vi "Create.vi"(8 "error in (no error)":errorcluster, 11 "NotifierMessenger in":refnum<class "NotifierMessenger.lvclass">) -> (0 "error out":errorcluster, 3 "NotifierMessenger out":refnum<class "NotifierMessenger.lvclass">)   [LabVIEW 2011, in "Messenging.lvlib" / "NotifierMessenger.lvclass"]
uses:
  NotifierMessenger.lvclass
  TextVarientMessage/MSG.lvclass
  NotifierMessenger.lvclass/NotifierMessenger.ctl
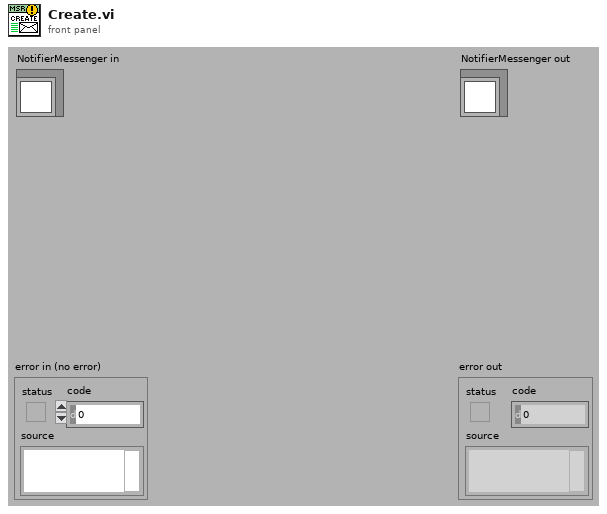
[diagram p1: front panel]
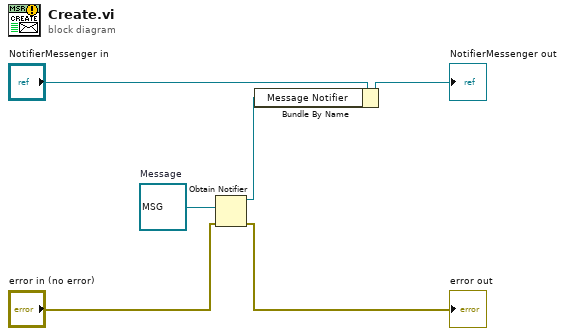
[diagram p0: block diagram]
diagram:
  w6 = refnum<class "MSG.lvclass"> refnum  # Message
  n1 = Obtain Notifier(notification data type=w6, error in (no error)="error in (no error)") -> (notifier out=w3:refnum<notifier>, error out=→"error out":errorcluster)  [unwired: 1 in, 2 out]
  n2 = Bundle By Name(cluster="NotifierMessenger in", "Message Notifier"=w3) -> (→"NotifierMessenger out":refnum<class "NotifierMessenger.lvclass">)
